vi "Override Empty Wheel Name_Multiple.vi"(8 "error in (no error)":errorcluster, 10 "wheel names":string[](array[string]), 11 "wheels in":refnum<class "NI_Robotics_Wheel.lvclass">[](array[class])) -> (0 "error out":errorcluster, 3 "wheels out":refnum<class "NI_Robotics_Wheel.lvclass">[](array[class]))   [LabVIEW 2017, in "NI_Robotics_Wheel.lvclass"]
uses:
  <vilib>/robotics/Steering/Wheel/NI_Robotics_Wheel.lvclass
  <vilib>/robotics/Steering/Wheel/NI_Robotics_Wheel.lvclass/NI_Robotics_Wheel.ctl
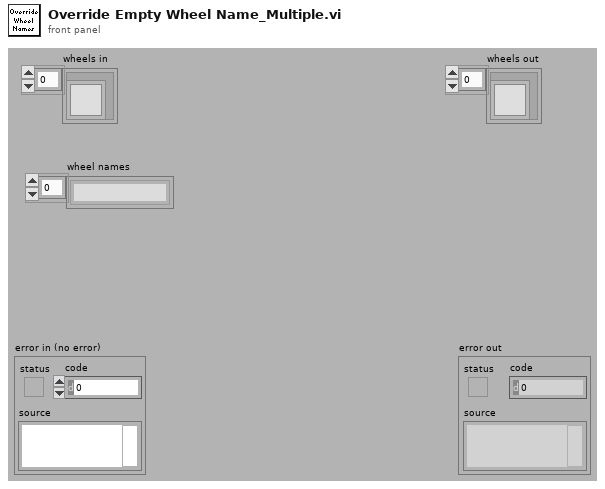
[diagram p1: front panel]
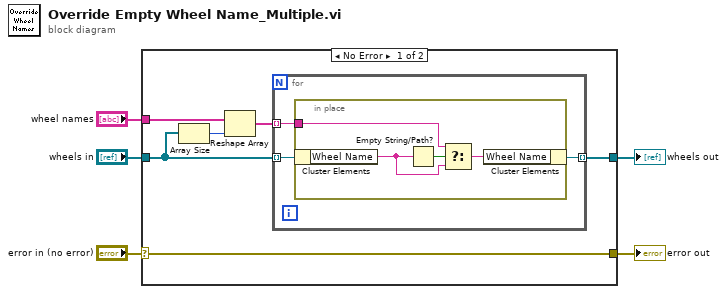
[diagram p0: block diagram]
diagram:
  n1 = case shown="No Error" "error in (no error)" {
    selector: "error in (no error)" -> [w11 w20]
    tunnel: [w11 w20] -> w4
    tunnel: "wheels in" -> [w7 w19]
    tunnel: "wheel names" -> [w9 _]
    tunnel: [w6 w19] -> w1
    frame No Error {
      n2 = Array Size(array=w7) -> (size(s)=w10:i32)
      n3 = Reshape Array(w9, w10) -> (w8:string[])
      n4 = for {
        tunnel: w8 -> [w13] mode=indexing
        tunnel: w7 -> [w14] mode=indexing
        tunnel: [w12] -> w6 mode=indexing
        n5 = in-place {
          in-place-border: w13 -> [w17]
          n6 = in-place-cluster #1(w14) -> ("Wheel Name"=w16:string)
          n7 = Empty String/Path?(string/path=w16) -> (empty?=w18:bool)
          n8 = Select(t=w17, s=w18, f=w16) -> (s? t:f=w15:string)
          n9 = in-place-cluster #1("Wheel Name"=w15) -> (w12:refnum<class "NI_Robotics_Wheel.lvclass">)
        }
      }
    }
    frame Error {
    }
  }
  "error out" <- w4
  "wheels out" <- w1
